vi "Name Test.vi"() -> ()   [LabVIEW 2020, in "Stream-TCP.lvlib"]
uses:
  Stream-TCP.lvlib
  Cleanup.vi
  TCP Server.lvclass
panel:
  out "VI Name":string
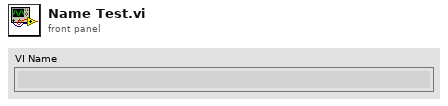
[diagram p1: front panel]
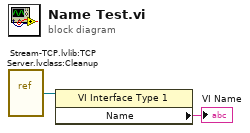
[diagram p0: block diagram]
diagram:
  n1 = vi-ref "Stream-TCP.lvlib:TCP Server.lvclass:Cleanup.vi"() -> (w2:refnum<vi>)
  n2 = property class="VI Interface Type 1"(reference=w2) -> ("Name"=→"VI Name":string)  [unwired: 1 in, 2 out]
